vi "Update_UI_ROI_List.vi"(8 "error in (no error)":errorcluster, 11 "LstBox Refnum":refnum<vi>) -> (0 "error out":errorcluster)   [LabVIEW 2019]
uses:
  Controls/ROI_List_Action.ctl
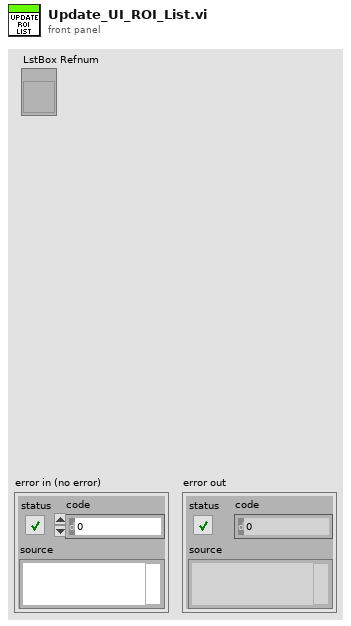
[diagram p1: front panel]
types:
  T1 = typedef "ROI_List_Action.ctl" = enum16{"Init", "Add ROI", "Delete ROI", "Get All ROI", "Get Specific ROI", "Set Analysis Setting", "Set Process Setting", "Replace All Entries", "ROIEntryBackup", "ROIEntryBackupClear", "ROIEntryReturn"}
  T2 = typedef "Vision_DataEntry.ctl" = cluster{"vROIName":string, "vROIContour":cluster{"Contour Type":u32, "ROI Type":u32, "Points":i32[]}, "ProcessSetting":T3[], "Analysis_Setting":T5}
  T3 = typedef "Process_Setting.ctl" = cluster{"Enum_PreProcess":T4, "Parameter":string}
  T4 = typedef "VisionProcessName.ctl" = enum16{"*CamParameter*", "CamAttributes", "*Preprocess*", "CG_Brightness", "C_Plane Extraction", "C_Threshold", "G_Lookup Table", "G_Threshold"}
  T5 = typedef "Analysis_Setting.ctl" = cluster{"PreProcess":T6, "Parameter":string}
  T6 = typedef "V_Analysis_Type.ctl" = enum16{"None", "C_Color Pattern Matching", "G_PatternMatching", "G_ShapeDectect", "G_GeometricMatch", "B_Area Check"}
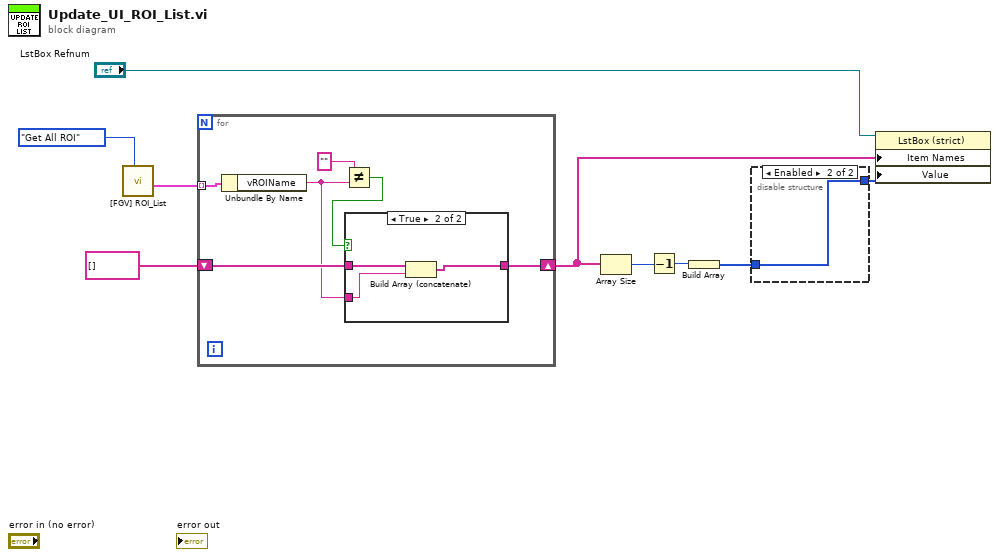
[diagram p0: block diagram]
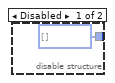
[diagram p2: hidden frame]
diagram:
  n1 = call "[FGV] ROI_List.vi"("Action"=ROI_List_Action."Get All ROI") -> ("All ROI"=w8:T2[])  [unwired: 8 in, 2 out]
  n2 = for {
    tunnel: w8 -> [w15] mode=indexing
    shift-right: [w10] -> w4
    shift-left: string[] [] -> [w12]
    n3 = Unbundle By Name(w15) -> ("vROIName"=w11:string)
    n4 = Not Equal?(x="", y=w11) -> (x != y?=w13:bool)
    n5 = case shown="True" w13 {
      tunnel: w12 -> [w16 w19]
      tunnel: w11 -> [_ w18]
      tunnel: [w16 w17] -> w10
      frame False {
      }
      frame True {
        n6 = Build Array (concatenate)(w19, w18) -> (w17:string[])
      }
    }
  }
  n7 = Array Size(array=w4) -> (size(s)=w3:i32)
  n8 = Decrement(x=w3) -> (x-1=w2:i32)
  n9 = Build Array(w2) -> (w1:i32[])
  n10 = disable-structure shown="Enabled" {
    disable-tunnel: [i32[] [] ("Value") w21] -> w5
    disable-tunnel: w1 -> [_ w21]
    frame Disabled {
    }
    frame Enabled {
    }
  }
  n11 = property class="LstBox (strict)"(reference="LstBox Refnum", "Item Names"=w4, "Value"=w5) -> ()  [unwired: 1 in, 2 out]
